vi "End stream Send.vi"(8 "error in":errorcluster, 11 "Call ID in":T2) -> (0 "error out":errorcluster, 1 "errorDetails":T1)   [LabVIEW 2021, in "streamtest_client.lvlib"]
uses:
  streamtest_client.lvlib
  <vilib>/gRPC/LabVIEW gRPC Library/grpc-lvsupport-release.lvlib
  <vilib>/gRPC/LabVIEW gRPC Library/Shared/grpcId.ctl
  Optimized Streaming/typedef/Call ID.ctl
  <vilib>/gRPC/LabVIEW gRPC Library/Shared/Any.ctl
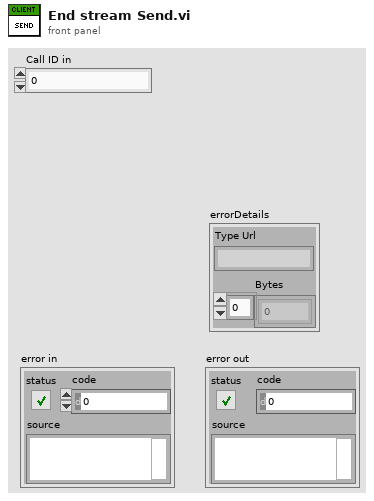
[diagram p1: front panel]
types:
  T1 = typedef "grpc-lvsupport-release.lvlib/Any.ctl" = cluster{"Type Url":string, "Bytes":u8[]}
  T2 = typedef "grpc-lvsupport-release.lvlib/grpcId.ctl" = u64
  T3 = typedef "Call ID.ctl" = cluster{"Call Id":T2, "occurrence":refnum<k4>}
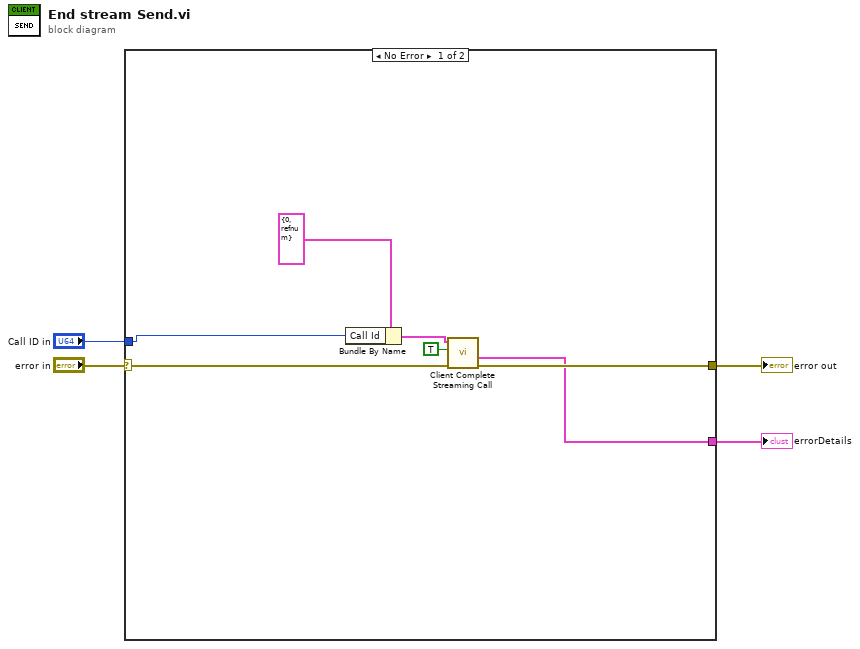
[diagram p0: block diagram]
diagram:
  n1 = case shown="No Error" "error in" {
    selector: "error in" -> [w11 w12]
    tunnel: [w10 w12] -> w3
    tunnel: "Call ID in" -> [w6 _]
    tunnel: [w9 _] -> w1
    frame No Error {
      n2 = Bundle By Name(cluster=T3 {"Call Id"=0, "occurrence"=refnum} ("Optimized Streaming in"), "Call Id"=w6) -> (w5:T3)
      n3 = call <vilib>:"Client Complete Streaming Call.vi"("error in"=w11, "Cancel All Reads (T)"=TRUE ("Cancel All Reads (F)"), "Optimized Streaming in"=w5) -> ("error out"=w10:errorcluster, "errorDetails"=w9:T1)  [unwired: 7 in]
    }
    frame Error {
    }
  }
  "error out" <- w3
  "errorDetails" <- w1
